vi "Process-error.vi"(8 "error in (no error)":errorcluster, 11 "ModComm in":T1) -> (0 "error out":errorcluster, 3 "ModComm out":T1)   [LabVIEW 2013, in "Server.lvlib" / "Server.lvclass"]
uses:
  Server.lvclass
  Object-reference.ctl
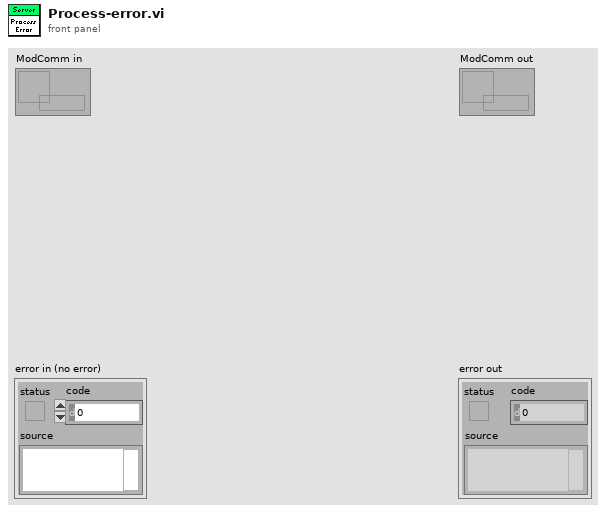
[diagram p1: front panel]
types:
  T1 = typedef "Server.lvlib/Server.lvclass/Object-reference.ctl" = refnum<data-value>
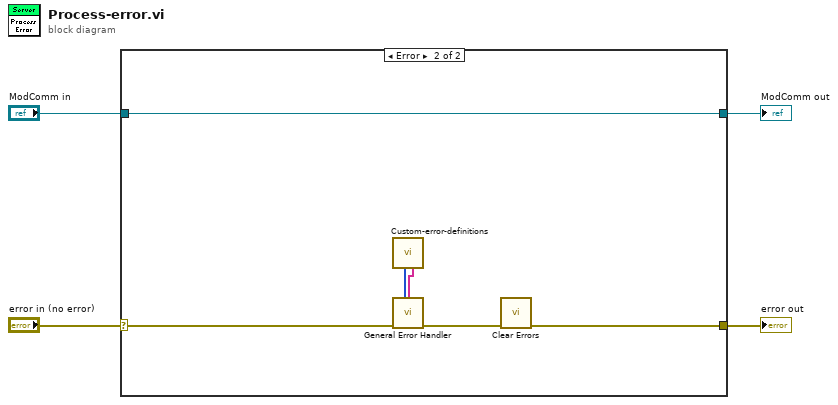
[diagram p0: block diagram]
diagram:
  n1 = case shown="Error" "error in (no error)" {
    selector: "error in (no error)" -> [w6 w12]
    tunnel: [w6 w9] -> w3
    tunnel: [w5 w11] -> w1
    tunnel: "ModComm in" -> [w5 w11]
    frame No Error {
    }
    frame Error {
      n2 = call "Custom-error-definitions.vi"() -> ("Descriptions"=w7:string[], "Error codes"=w8:i32[])  [unwired: 9 in, 1 out]
      n3 = call <vilib>:"General Error Handler.vi"("[user-defined codes]"=w8, "[user-defined descriptions]"=w7, "error in (no error)"=w12) -> ("error out"=w10:errorcluster)  [unwired: 8 in, 4 out]
      n4 = call <vilib>:"Clear Errors.vi"("error in (no error)"=w10) -> ("error out"=w9:errorcluster)  [unwired: 6 in]
    }
  }
  "error out" <- w3
  "ModComm out" <- w1
